vi "Main.vi"(11 "Module Admin":refnum<class "Delacor_lib_QMH_Module Admin.lvclass">) -> ()   [LabVIEW 2019, in "Dashboard.lvlib"]
doc: "This template is based off of the Queued Message Handler design pattern and the Queued Message Handler project template that ships with LabVIEW.\n\nThe main difference is that the queue is private to this module and communication between modules is performed via Broadcast and Request events.\n\nRequest events are wrapped in public API methods and are handled in the Event Handling Loop (EHL) of this VI. Any module can register for Broadcast events sent by this module. The EHL generates messages based on user interface actions.\n\nThe Message Handling Loop (MHL) processes messages generated by the EHL, or by other messages. The messages are string values, so new messages can be added easily to the Message Cases case structure in the MHL. Each message cluster can also provide an optional value for Message Data, which is a variant that can be converted to whatever message-specific data is required.\n_____\nBased on Delacor QMH Project Template 5.0.0.82."
uses:
  Dashboard.lvlib
  <vilib>/Delacor/Delacor QMH/Libraries/Module Admin_class/Delacor_lib_QMH_Module Admin.lvclass
  picam32_LabView_SDK/PICam_lib/types/PicamGatingMode.ctl
  picam32_LabView_SDK/PICam_lib/types/PicamPulse.ctl
  picam32_LabView_SDK/PICam_lib/Ctrls/PicamAdcAnalogGain.ctl
  picam32_LabView_SDK/PICam_lib/Ctrls/PicamAdcQuality.ctl
  picam32_LabView_SDK/PICam_lib/types/PicamSensorTemperatureStatus.ctl
  Module Data--cluster.ctl
  Utility/Types/SetOrGet.ctl
  Update Image Argument--cluster.ctl
  <vilib>/Delacor/Delacor QMH/Libraries/Message Queue_class/Delacor_lib_QMH_Message Queue.lvclass/Delacor_lib_QMH_Message Queue.ctl
  Stop Argument--cluster.ctl
  <vilib>/Utility/miscctls.llb/LVPointTypeDef.ctl
  <vilib>/Delacor/Delacor QMH/Libraries/Module Admin_class/Delacor_lib_QMH_Module Admin.lvclass/Delacor_lib_QMH_Module Admin.ctl
  <vilib>/Delacor/Delacor QMH/Libraries/Message Queue_class/Delacor_lib_QMH_Enqueue Message (Single).vi
  <vilib>/Delacor/Delacor QMH/Libraries/Module Admin_class/Delacor_lib_QMH_Get External Launch.vi
  <vilib>/Utility/error.llb/Error Cluster From Error Code.vi
  <vilib>/ErrorRing/Error Ring.xnode
  <vilib>/Delacor/Delacor QMH/Libraries/Message Queue_class/Delacor_lib_QMH_Message Queue.lvclass
  Spectrometer/Spectrometer.lvlib
  Camera/Camera.lvlib
  FileIO/FileIO.lvlib
  Acquisition Example/Acquisition Example.lvlib
  Notification/Notification.lvlib
  picam32_LabView_SDK/PICam_lib/PICam.lvlib
panel:
  out "Is Running FileIO":bool
  out "Is Running Notification":bool
  in  "Stop Module Notification":bool
  in  "Start Module Notification":bool
  out "Waveform Chart":dbl(graph)
  in  "Acquisition VIs":enum16{"Acquisition Example"}(ring)
  in  "Start Acquisition VI":bool
  in  "Device Tabs":enum32{"Spectrometer", "Camera"}(tab)
  in  "Set Grating":bool
  in  "Set Slit Width":bool
  in  "Grating":i32
  in  "Slit Width":dbl
  in  "Set Wavelength":bool
  in  "Wavelength":dbl
  in  "Tab Control - Camera Parameters":T1(tab)
  in  "IntensifierGain":i32
  in  "EMIccdGain":i32
  in  "CorrectPixelBias":bool
  in  "AdcSpeed":dbl
  in  "AdcBitDepth":i32
  in  "PicamAdcQuality":T2=enum."LowNoise"
  in  "AdcAnalogGain":T3=enum."Medium"
  in  "AdcEMGain":i32
  out "SensorTemperatureStatus":T4
  in  "SensorTemperatureSetPoint":dbl
  out "SensorTemperatureReading":dbl
  out "Temperature Chart":dbl(graph)
  in  "RepetitiveGate":T5
  in  "GatingMode":T6
  in  "V Binning":i32
  in  "V Width":i32
  in  "Vertical":i32
  in  "H Binning":i32
  in  "H Width":i32
  in  "Horizontal":i32
  in  "Acquire Continuously":bool
  in  "Set Accumulations":bool
  in  "Set ROI":bool
  in  "Accumulations":i64 min=0 step=1
  out "Spectrum Graph":u16[][](graph)
  out "CCD Image":u16[][](graph)
  out "Is Running Camera":bool
  in  "Stop Module Camera":bool
  in  "Start Module Camera":bool
  out "Is Running Spectrometer":bool
  in  "Stop Module Spectrometer":bool
  in  "Start Module Spectrometer":bool
  out "Status":string
  # "Module Status"
  # "Spectrometer"
  # "Camera"
  # "Notification"
  # "FileIO"
  # "Data Acquisition"
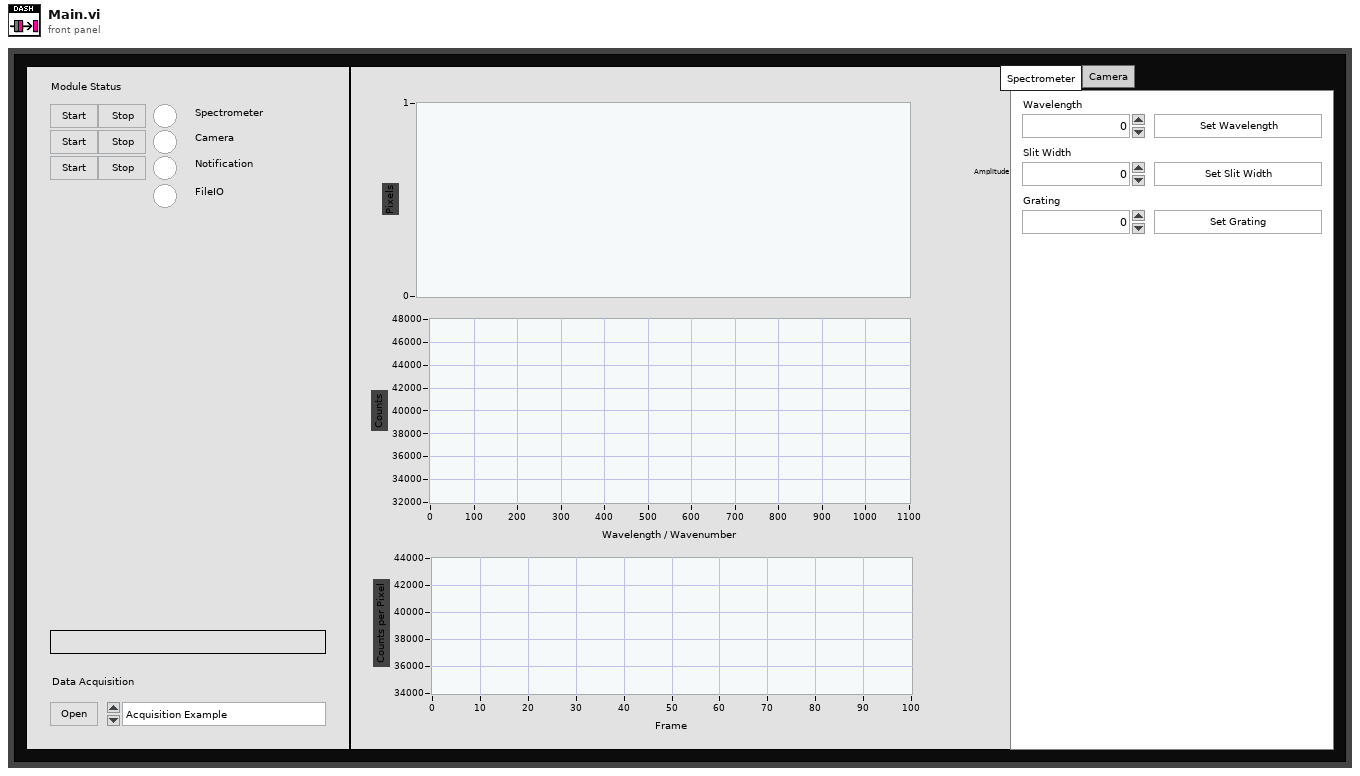
[diagram p1: front panel]
types:
  T1 = enum32{"Intensifier", "ADC", "Gating", "Temperature"}
  T2 = typedef "PICam.lvlib/PicamAdcQuality.ctl" = enum16{"None", "LowNoise", "HighCapacity", "ElectronMultiplied", "HighSpeed"}
  T3 = typedef "PICam.lvlib/PicamAdcAnalogGain.ctl" = enum16{"None", "Low", "Medium", "High"}
  T4 = typedef "PICam.lvlib/PicamSensorTemperatureStatus.ctl" = enum16{"None", "Unlocked", "Locked", "Faulted"}
  T5 = typedef "PICam.lvlib/PicamPulse.ctl" = cluster{"delay":dbl, "width":dbl}
  T6 = typedef "PICam.lvlib/PicamGatingMode.ctl" = enum16{"None", "Repetitive", "Sequential", "Custom", "Disabled"}
  T7 = typedef "Dashboard.lvlib/Request Events--cluster.ctl" = cluster{"Stop Module":refnum<user-event>, "Show Panel":refnum<user-event>, "Hide Panel":refnum<user-event>, "Get Module Execution Status":refnum<user-event>, "Show Diagram":refnum<user-event>}
  T8 = typedef "Notification.lvlib/Broadcast Events--cluster.ctl" = cluster{"Module Did Init":refnum<user-event>, "Status Updated":refnum<user-event>, "Error Reported":refnum<user-event>, "Module Did Stop":refnum<user-event>, "Update Module Execution Status":refnum<user-event>}
  T9 = typedef "Spectrometer.lvlib/Broadcast Events--cluster.ctl" = cluster{"Module Did Init":refnum<user-event>, "Status Updated":refnum<user-event>, "Error Reported":refnum<user-event>, "Module Did Stop":refnum<user-event>, "Update Module Execution Status":refnum<user-event>, "Broadcast Wavelength":refnum<user-event>, "Broadcast Slit Width":refnum<user-event>, "Broadcast Grating":refnum<user-event>}
  T10 = typedef "Camera.lvlib/Broadcast Events--cluster.ctl" = cluster{"Module Did Init":refnum<user-event>, "Status Updated":refnum<user-event>, "Error Reported":refnum<user-event>, "Module Did Stop":refnum<user-event>, "Update Module Execution Status":refnum<user-event>, "Broadcast Image":refnum<user-event>, "Broadcast Exposure Time":refnum<user-event>, "Broadcast Binning":refnum<user-event>, "Broadcast GatingMode":refnum<user-event>, "Broadcast RepetitiveGate":refnum<user-event>, "Broadcast IntensifierStatus":refnum<user-event>, "Broadcast IntensifierGain":refnum<user-event>, "Broadcast EMIccdGainControlMode":refnum<user-event>, "Broadcast EMIccdGain":refnum<user-event>, "Broadcast FloatingPoint Parameter":refnum<user-event>, "Broadcast Integer Parameter":refnum<user-event>, "Broadcast LargeInteger Parameter":refnum<user-event>, "Broadcast Pulse Parameter":refnum<user-event>, "Broadcast SensorTemperatureStatus":refnum<user-event>}
  T11 = typedef "FileIO.lvlib/Broadcast Events--cluster.ctl" = cluster{"Module Did Init":refnum<user-event>, "Status Updated":refnum<user-event>, "Error Reported":refnum<user-event>, "Module Did Stop":refnum<user-event>, "Update Module Execution Status":refnum<user-event>, "File Prepared":refnum<user-event>, "Wrote to File":refnum<user-event>}
  T12 = typedef "Dashboard.lvlib/Module Data--cluster.ctl" = cluster{"Status":string, "Image":u16[][]}
  T13 = enum32{"Invalid", "Standard", "Closed", "Hidden", "Minimized", "Maximized"}
  T14 = typedef "SetOrGet.ctl" = enum16{"Set", "Get"}
  T15 = typedef "Dashboard.lvlib/Update Image Argument--cluster.ctl" = cluster{"Image":u16[][]}
  T16 = enum32{"invalid lock state", "Not Locked", "Locked (No Password)", "Password-protected"}
  T17 = typedef "Dashboard.lvlib/Stop Argument--cluster.ctl" = cluster{"Origin":string, "Exit via Stop Module Req?":bool, "Wait for Module to stop?":bool}
  T18 = typedef "LVPointTypeDef.ctl" = cluster{"Horizontal":i16, "Vertical":i16}
  T19 = typedef "Camera.lvlib/Set GatingMode (Reply Payload)--cluster.ctl" = cluster{"PicamGatingMode":T6, "Set GatingMode_error":errorcluster}
  T20 = typedef "Camera.lvlib/Set RepetitiveGate (Reply Payload)--cluster.ctl" = cluster{"RepetitiveGate":T5, "Set RepetitiveGate_error":errorcluster}
  T21 = typedef "Camera.lvlib/Set Accumulations (Reply Payload)--cluster.ctl" = cluster{"Accumulations":i64, "Set Accumulations_error":errorcluster}
  T22 = cluster{"Horizontal":i32, "H Width":i32, "H Binning":i32, "Vertical":i32, "V Width":i32, "V Binning":i32}
  T23 = typedef "Spectrometer.lvlib/Set Slit Width (Reply Payload)--cluster.ctl" = cluster{"Slit Width (um)":dbl, "Set Slit Width_error":errorcluster}
  T24 = typedef "Spectrometer.lvlib/Set Wavelength (Reply Payload)--cluster.ctl" = cluster{"Wavelength":dbl, "Set Wavelength_error":errorcluster}
  T25 = typedef "Camera.lvlib/SetGet Integer Parameter (Reply Payload)--cluster.ctl" = cluster{"PicamParameter":T26, "Integer Value":i32, "SetGet Integer Parameter_error":errorcluster}
  T26 = typedef "PICam.lvlib/PicamParameter.ctl" = i32
  T27 = typedef "Camera.lvlib/SetGet FloatingPoint Parameter (Reply Payload)--cluster.ctl" = cluster{"FloatingPoint Value":dbl, "PicamParameter":T26, "SetGet FloatingPoint Parameter_error":errorcluster}
  T28 = typedef "Camera.lvlib/ROI--cluster.ctl" = cluster{"_Horizontal":i32, "_Horizontal Width":i32, "_Horizontal Binning":i32, "_Vertical":i32, "_Vertical Width":i32, "_Vertical Binning":i32}
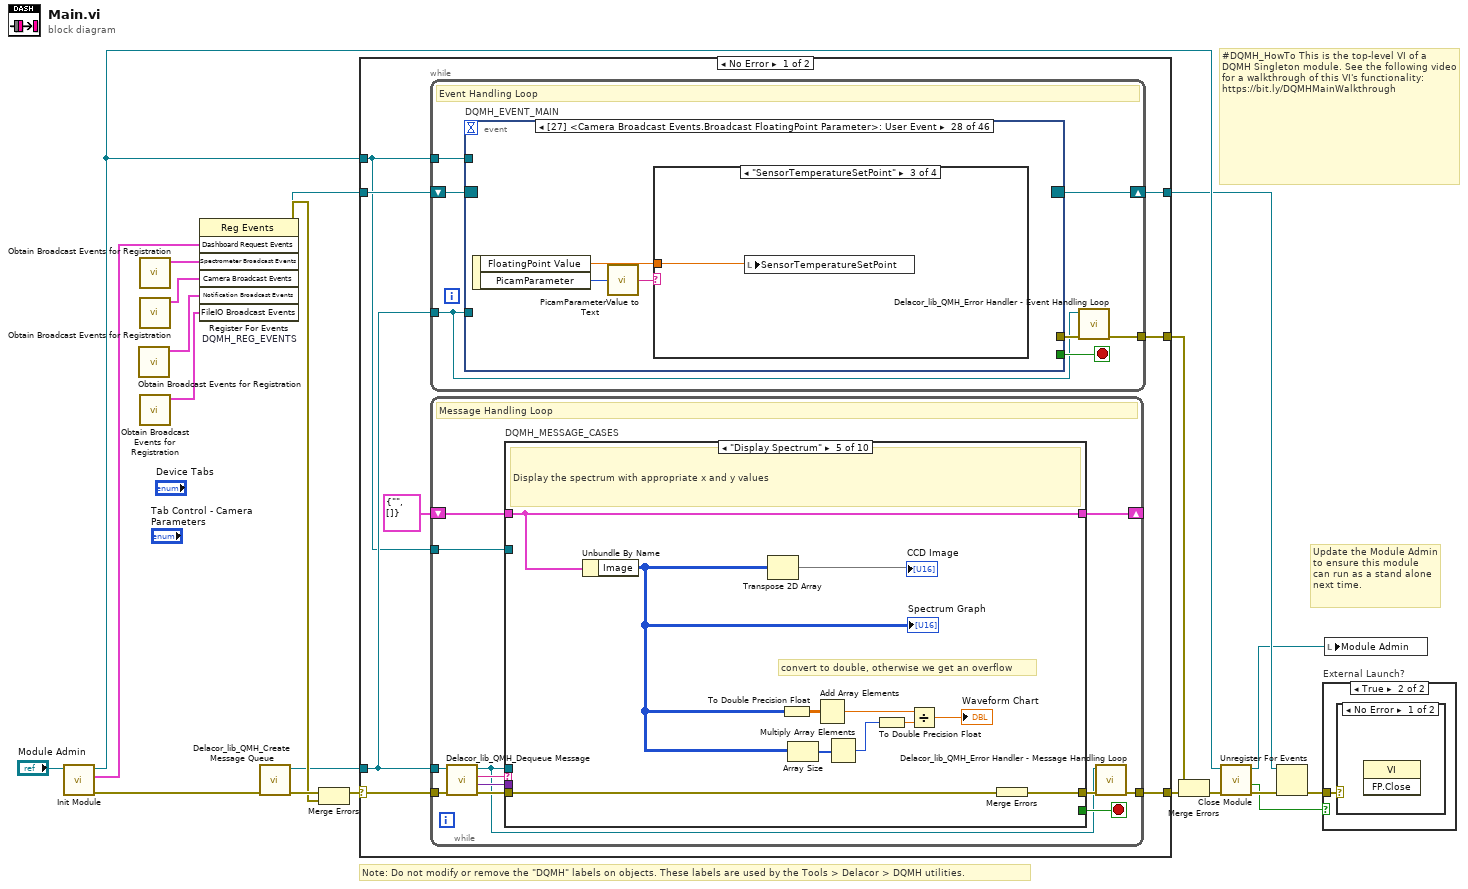
[diagram p0: block diagram]
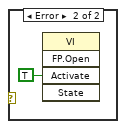
[diagram p3: hidden frame]
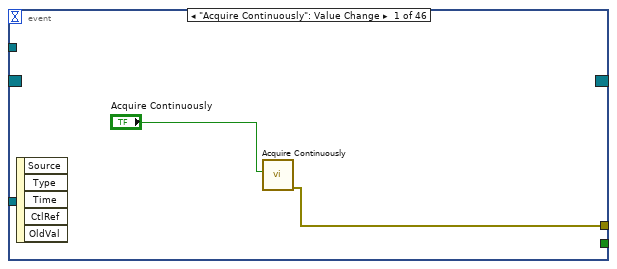
[diagram p4: hidden frame]
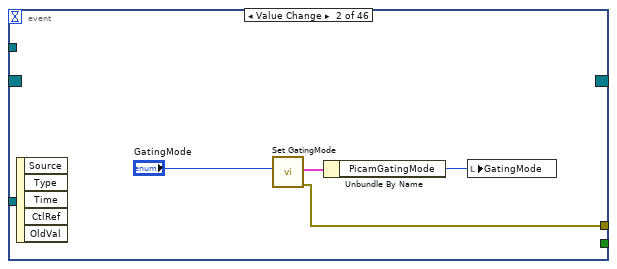
[diagram p5: hidden frame]
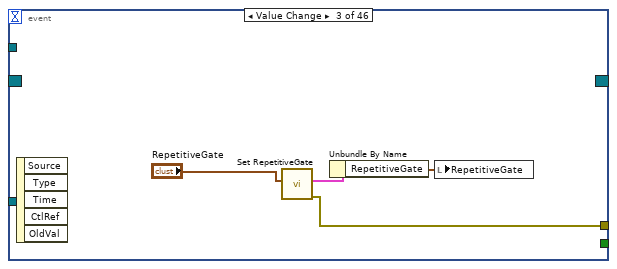
[diagram p6: hidden frame]
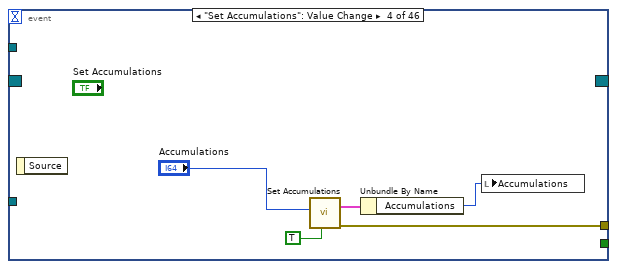
[diagram p7: hidden frame]
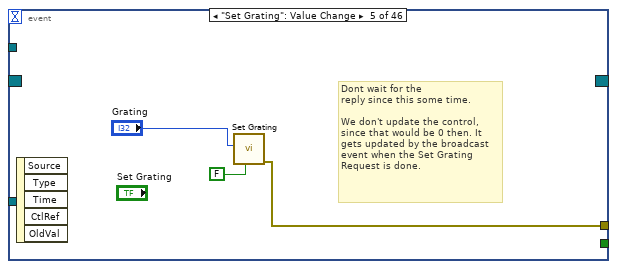
[diagram p8: hidden frame]
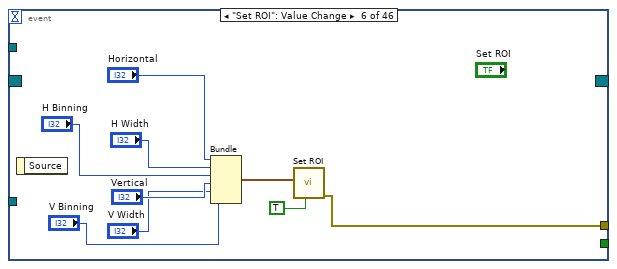
[diagram p9: hidden frame]
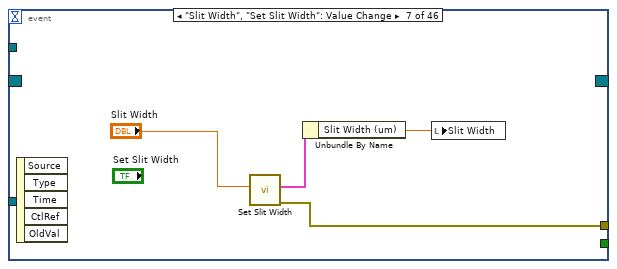
[diagram p10: hidden frame]
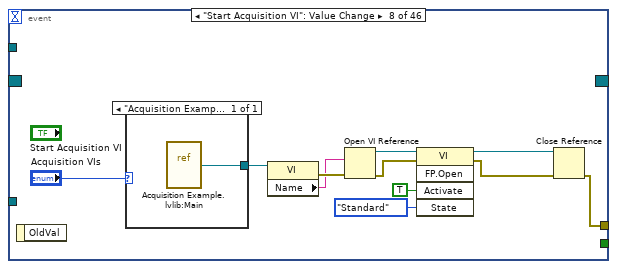
[diagram p11: hidden frame]
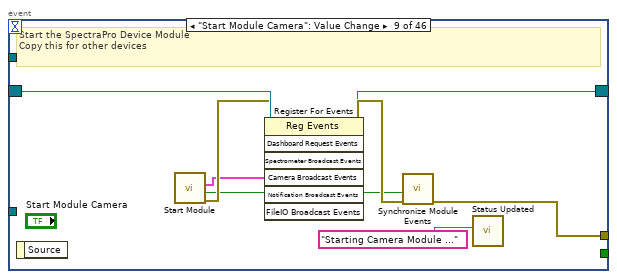
[diagram p12: hidden frame]
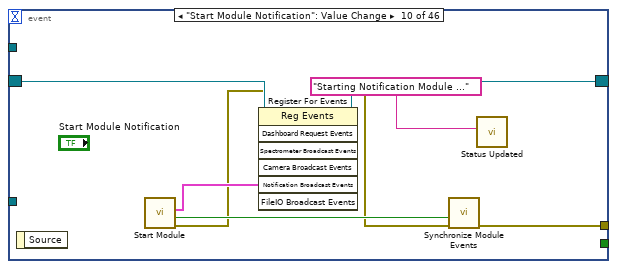
[diagram p13: hidden frame]
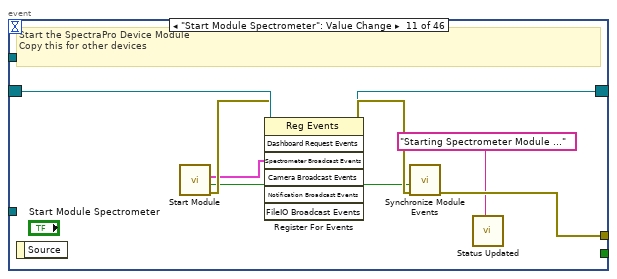
[diagram p14: hidden frame]
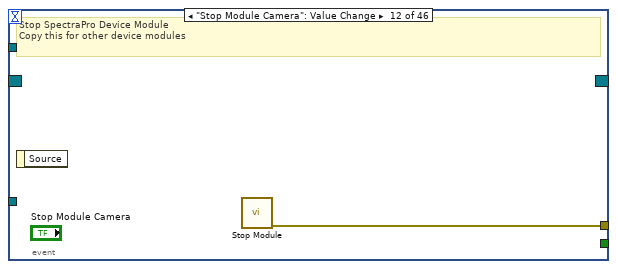
[diagram p15: hidden frame]
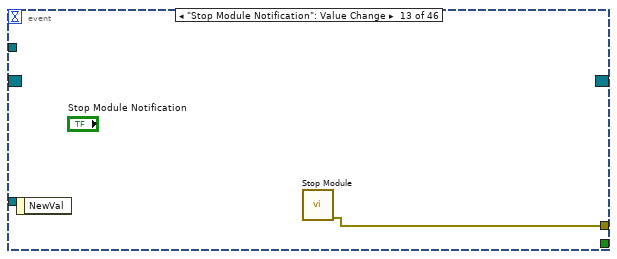
[diagram p16: hidden frame]
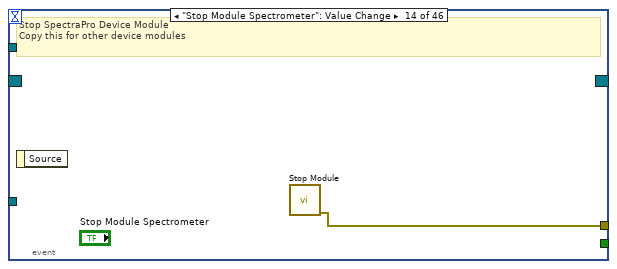
[diagram p17: hidden frame]
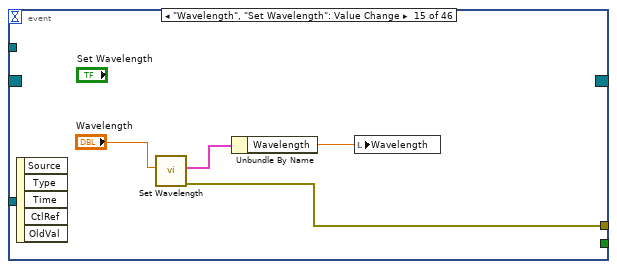
[diagram p18: hidden frame]
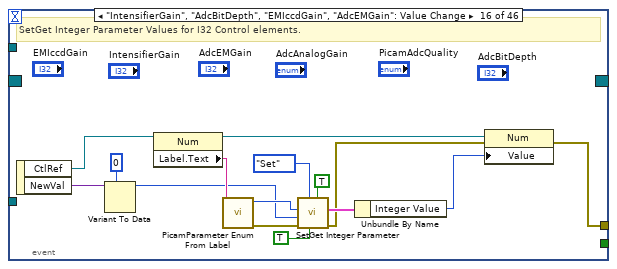
[diagram p19: hidden frame]
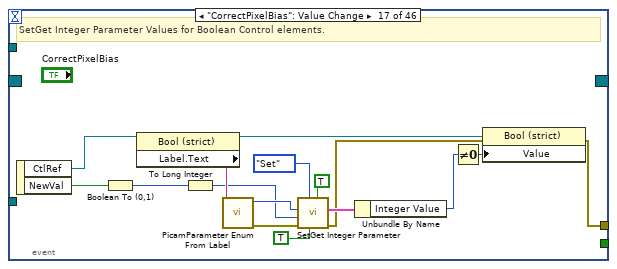
[diagram p20: hidden frame]
diagram:
  # "#DQMH_HowTo This is the top-level VI of a DQMH Singleton module. See the following video for a walkthrough of this VI's functionality: https://bit.ly/DQMHMainWalkthrough"
  # "Note: Do not modify or remove the \"DQMH\" labels on objects. These labels are used by the Tools > Delacor > DQMH utilities."
  # "Update the Module Admin to ensure this module can run as a stand alone next time."
  n1 = call "Init Module.vi"("Singleton Module Admin in"="Module Admin") -> ("error out"=w20:errorcluster, "Dashboard Request Events"=w9:T7, "Singleton Module Admin out"=w12:refnum<class "Delacor_lib_QMH_Module Admin.lvclass">)  [unwired: 8 in]
  n2 = call "Obtain Broadcast Events for Registration.vi"() -> ("Notification Broadcast Events"=w1:T8)  [unwired: 9 in, 2 out]
  n3 = call "Obtain Broadcast Events for Registration.vi"() -> ("Spectrometer Broadcast Events"=w4:T9)  [unwired: 9 in, 2 out]
  n4 = call "Obtain Broadcast Events for Registration.vi"() -> ("Camera Broadcast Events"=w3:T10)  [unwired: 9 in, 2 out]
  n5 = call "Obtain Broadcast Events for Registration.vi"() -> ("FileIO Broadcast Events"=w2:T11)  [unwired: 9 in, 2 out]
  n6 = register-events "DQMH_REG_EVENTS"(w9, w4, w3, w1, w2) -> (reference out=w10:refnum<event-registration>, error out=w13:errorcluster)  [unwired: 2 in]
  n7 = call <vilib>:"Delacor_lib_QMH_Create Message Queue.vi"("error in (no error)"=w20) -> ("error out"=w15:errorcluster, "Message Queue"=w8:refnum<class "Delacor_lib_QMH_Message Queue.lvclass">)  [unwired: 9 in]
  n8 = Merge Errors(w15, w13) -> (w14:errorcluster)
  n9 = case shown="No Error" w14 {
    selector: w14 -> [w27 w357]
    tunnel: [w29 w356] -> w21
    tunnel: [w26 w362] -> w11
    tunnel: w10 -> [w24 w362]
    tunnel: w8 -> [w23 w355]
    tunnel: [w28 _] -> w18
    tunnel: w12 -> [w22 w358]
    frame No Error {
      n10 = while {
        tunnel: w23 -> [w30]
        shift-right: [w33] -> w26
        shift-left: w24 -> [w34]
        tunnel: [w35] -> w28
        tunnel: w22 -> [w31]
        stop <- w32 stop-if-true
        # "Event Handling Loop"
        n11 = event "DQMH_EVENT_MAIN" shown="[27] <Camera Broadcast Events.Broadcast FloatingPoint Parameter>: User Event" {
          selector: w34 -> [_ _ _ _ _ _ _ _ w87 w93 w103 _ _ _ _ _ _ _ _ _ _ _ _ _ _ _ _ _ _ _ _ _ _ _ _ _ _ _ _ _ _ _ _ _ _ _]
          dyn-events: [_ _ _ _ _ _ _ _ w84 w92 w97 _ _ _ _ _ _ _ _ _ _ _ _ _ _ _ _ _ _ _ _ _ _ _ _ _ _ _ _ _ _ _ _ _ _ _] -> w33
          timeout: _ -> [_ _ _ _ _ _ _ _ _ _ _ _ _ _ _ _ _ _ _ _ _ _ _ _ _ _ _ _ _ _ _ _ _ _ _ _ _ _ _ _ _ _ _ _ _ _]
          tunnel: [_ _ _ _ _ _ _ _ _ _ _ _ _ _ _ _ _ _ _ _ _ _ _ _ _ _ _ _ _ _ _ _ TRUE ("Discard?") _ _ _ _ _ _ _ _ _ _ _ _ _] -> w32
          tunnel: w30 -> [_ _ _ _ _ _ _ _ _ _ _ _ _ _ _ _ _ _ _ _ _ w173 _ _ _ _ _ _ _ _ _ _ w215 _ _ _ _ _ _ _ _ _ _ _ _ w234]
          tunnel: [w37 w41 w45 w50 w53 w63 w66 w74 w82 w94 w101 w104 w105 w106 w109 w113 w129 w144 _ _ _ w174 _ _ _ _ _ _ w194 _ _ _ w218 _ _ _ _ _ _ _ _ _ _ _ _ w236] -> w36
          tunnel: w31 -> [_ _ _ _ _ _ _ _ _ _ _ _ _ _ _ _ _ _ _ _ _ _ _ _ _ _ _ _ _ _ _ _ _ _ _ _ _ _ _ _ _ _ _ _ _ _]
          event "Acquire Continuously": Value Change {
            n12 = event-data() -> ()  [unwired: 1 in, 5 out]
            n13 = call "Acquire Continuously.vi"("Acquire Continuously"="Acquire Continuously") -> ("error out"=w37:errorcluster)  [unwired: 10 in]
          }
          event Value Change {
            n14 = event-data() -> ()  [unwired: 1 in, 5 out]
            n15 = call "Set GatingMode.vi"("PicamGatingMode"="GatingMode") -> ("error out"=w41:errorcluster, "Reply Payload"=w40:T19)  [unwired: 8 in, 1 out]
            n16 = Unbundle By Name(w40) -> ("PicamGatingMode"=w39:T6)
            n17 = local write "GatingMode"(w39) -> ()
          }
          event Value Change {
            n18 = event-data() -> ()  [unwired: 1 in, 5 out]
            n19 = call "Set RepetitiveGate.vi"("RepetitiveGate"="RepetitiveGate") -> ("error out"=w45:errorcluster, "Reply Payload"=w44:T20)  [unwired: 8 in, 1 out]
            n20 = Unbundle By Name(w44) -> ("RepetitiveGate"=w43:T5)
            n21 = local write "RepetitiveGate"(w43) -> ()
          }
          event "Set Accumulations": Value Change {
            n22 = event-data() -> ()  [unwired: 1 in, 1 out]
            n23 = call "Set Accumulations.vi"("wait for reply (T)"=TRUE, "Accumulations"="Accumulations") -> ("error out"=w50:errorcluster, "Reply Payload"=w48:T21)  [unwired: 7 in, 1 out]
            n24 = Unbundle By Name(w48) -> ("Accumulations"=w47:i64)
            n25 = local write "Accumulations"(w47) -> ()
          }
          event "Set Grating": Value Change {
            # "Dont wait for the\nreply since this some time.\n\nWe don't update the control,\nsince that would be 0 then. It\ngets updated by the broadcast\nevent when the Set Grating\nRequest is done."
            n26 = event-data() -> ()  [unwired: 1 in, 5 out]
            n27 = call "Set Grating.vi"("wait for reply (T)"=FALSE, "Grating ID"="Grating") -> ("error out"=w53:errorcluster)  [unwired: 7 in, 2 out]
          }
          event "Set ROI": Value Change {
            n28 = event-data() -> ()  [unwired: 1 in, 1 out]
            n29 = Bundle("Horizontal"="Horizontal", "H Width"="H Width", "H Binning"="H Binning", "Vertical"="Vertical", "V Width"="V Width", "V Binning"="V Binning") -> (w55:T22)  [unwired: 1 in]
            n30 = call "Set ROI.vi"("wait for reply (T)"=TRUE, "ROI"=w55) -> ("error out"=w63:errorcluster)  [unwired: 7 in, 2 out]
          }
          event "Slit Width", "Set Slit Width": Value Change {
            n31 = event-data() -> ()  [unwired: 1 in, 5 out]
            n32 = call "Set Slit Width.vi"("Slit Width (um)"="Slit Width") -> ("error out"=w66:errorcluster, "Reply Payload"=w65:T23)  [unwired: 8 in, 1 out]
            n33 = Unbundle By Name(w65) -> ("Slit Width (um)"=w64:dbl)
            n34 = local write "Slit Width"(w64) -> ()
          }
          event "Start Acquisition VI": Value Change {
            n35 = event-data() -> ()  [unwired: 1 in, 1 out]
            n36 = case shown="\"Acquisition Example\", Default" "Acquisition VIs" {
              tunnel: [w79] -> w77
              frame "Acquisition Example", Default {
                n37 = vi-ref "Acquisition Example.lvlib:Main.vi"() -> (w79:refnum<vi>)
              }
            }
            n38 = property class="VI"(reference=w77) -> (error out=w76:errorcluster, "Name"=w75:string)  [unwired: 1 in, 1 out]
            n39 = Open VI Reference(vi path=w75, error in (no error)=w76) -> (vi reference=w73:refnum<vi>, error out=w70:errorcluster)  [unwired: 4 in]
            n40 = invoke class="VI" method="FP.Open"(reference=w73, error in=w70, "Activate"=TRUE ("Activate?"), "State"=T13."Standard") -> (reference out=w71:refnum<vi>, error out=w69:errorcluster)  [unwired: 1 in, 3 out]
            n41 = Close Reference(reference=w71, error in (no error)=w69) -> (error out=w74:errorcluster)
          }
          event "Start Module Camera": Value Change {
            # "Start the SpectraPro Device Module\nCopy this for other devices"
            n42 = event-data() -> ()  [unwired: 1 in, 1 out]
            n43 = call "Start Module.vi"() -> ("error out"=w83:errorcluster, "Wait for Event Sync?"=w80:bool, "Camera Broadcast Events"=w81:T10)  [unwired: 8 in, 1 out]
            n44 = register-events(reference=w87, error in=w83, w81) -> (reference out=w84:refnum<event-registration>, error out=w86:errorcluster)  [unwired: 4 in]
            n45 = call "Synchronize Module Events.vi"("error in (no error)"=w86, "Wait for Event Sync?"=w80) -> ("error out"=w82:errorcluster)  [unwired: 9 in]
            n46 = call "Status Updated.vi"("Status"="Starting Camera Module ...") -> ()  [unwired: 10 in, 1 out]
          }
          event "Start Module Notification": Value Change {
            n47 = event-data() -> ()  [unwired: 1 in, 1 out]
            n48 = call "Start Module.vi"() -> ("error out"=w90:errorcluster, "Wait for Event Sync?"=w95:bool, "Notification Broadcast Events"=w91:T8)  [unwired: 8 in, 1 out]
            n49 = register-events(reference=w93, error in=w90, w91) -> (reference out=w92:refnum<event-registration>, error out=w89:errorcluster)  [unwired: 4 in]
            n50 = call "Synchronize Module Events.vi"("error in (no error)"=w89, "Wait for Event Sync?"=w95) -> ("error out"=w94:errorcluster)  [unwired: 9 in]
            n51 = call "Status Updated.vi"("Status"="Starting Notification Module ...") -> ()  [unwired: 10 in, 1 out]
          }
          event "Start Module Spectrometer": Value Change {
            # "Start the SpectraPro Device Module\nCopy this for other devices"
            n52 = event-data() -> ()  [unwired: 1 in, 1 out]
            n53 = call "Start Module.vi"() -> ("error out"=w102:errorcluster, "Wait for Event Sync?"=w99:bool, "Spectrometer Broadcast Events"=w96:T9)  [unwired: 8 in, 1 out]
            n54 = register-events(reference=w103, error in=w102, w96) -> (reference out=w97:refnum<event-registration>, error out=w100:errorcluster)  [unwired: 4 in]
            n55 = call "Synchronize Module Events.vi"("error in (no error)"=w100, "Wait for Event Sync?"=w99) -> ("error out"=w101:errorcluster)  [unwired: 9 in]
            n56 = call "Status Updated.vi"("Status"="Starting Spectrometer Module ...") -> ()  [unwired: 10 in, 1 out]
          }
          event "Stop Module Camera": Value Change {
            # "Stop SpectraPro Device Module\nCopy this for other device modules"
            n57 = event-data() -> ()  [unwired: 1 in, 1 out]
            n58 = call "Stop Module.vi"() -> ("error out"=w104:errorcluster)  [unwired: 11 in]
          }
          event "Stop Module Notification": Value Change {
            n59 = event-data() -> ()  [unwired: 1 in, 1 out]
            n60 = call "Stop Module.vi"() -> ("error out"=w105:errorcluster)  [unwired: 11 in]
          }
          event "Stop Module Spectrometer": Value Change {
            # "Stop SpectraPro Device Module\nCopy this for other device modules"
            n61 = event-data() -> ()  [unwired: 1 in, 1 out]
            n62 = call "Stop Module.vi"() -> ("error out"=w106:errorcluster)  [unwired: 11 in]
          }
          event "Wavelength", "Set Wavelength": Value Change {
            n63 = event-data() -> ()  [unwired: 1 in, 5 out]
            n64 = call "Set Wavelength.vi"("Wavelength"="Wavelength") -> ("error out"=w109:errorcluster, "Reply Payload"=w108:T24)  [unwired: 8 in, 1 out]
            n65 = Unbundle By Name(w108) -> ("Wavelength"=w107:dbl)
            n66 = local write "Wavelength"(w107) -> ()
          }
          event "IntensifierGain", "AdcBitDepth", "EMIccdGain", "AdcEMGain": Value Change {
            # "SetGet Integer Parameter Values for I32 Control elements."
            n67 = event-data() -> ("CtlRef"=w122:refnum<vi>, "NewVal"=w125:variant)  [unwired: 1 in]
            n68 = Variant To Data(type=0, Variant=w125) -> (data=w111:i32)  [unwired: 1 in, 1 out]
            n69 = property class="Num"(reference=w122) -> (reference out=w117:refnum<vi>, "Label.Text"=w121:string)  [unwired: 1 in, 1 out]
            n70 = call "PicamParameter Enum From Label.vi"("String"=w121) -> ("error out"=w123:errorcluster, "Numeric"=w124:i32)  [unwired: 9 in]
            n71 = call "SetGet Integer Parameter.vi"("Broadcast"=TRUE, "wait for reply (T)"=TRUE, "SetOrGet"=SetOrGet."Set", "error in (no error)"=w123, "Integer Value"=w111, "PicamParameter"=w124) -> ("error out"=w114:errorcluster, "Reply Payload"=w116:T25)  [unwired: 3 in, 1 out]
            n72 = Unbundle By Name(w116) -> ("Integer Value"=w115:i32)
            n73 = property class="Num"(reference=w117, error in=w114, "Value"=w115) -> (error out=w113:errorcluster)  [unwired: 1 out]
          }
          event "CorrectPixelBias": Value Change {
            # "SetGet Integer Parameter Values for Boolean Control elements."
            n74 = event-data() -> ("CtlRef"=w138:refnum<vi>, "NewVal"=w141:bool)  [unwired: 1 in]
            n75 = Boolean To (0,1)(Boolean=w141) -> (0, 1=w128:i16)
            n76 = property class="Bool (strict)"(reference=w138) -> (reference out=w133:refnum<vi>, "Label.Text"=w137:string)  [unwired: 1 in, 1 out]
            n77 = To Long Integer(number=w128) -> (32bit integer=w127:i32)
            n78 = call "PicamParameter Enum From Label.vi"("String"=w137) -> ("error out"=w139:errorcluster, "Numeric"=w140:i32)  [unwired: 9 in]
            n79 = call "SetGet Integer Parameter.vi"("Broadcast"=TRUE, "wait for reply (T)"=TRUE, "SetOrGet"=SetOrGet."Set", "error in (no error)"=w139, "Integer Value"=w127, "PicamParameter"=w140) -> ("error out"=w130:errorcluster, "Reply Payload"=w132:T25)  [unwired: 3 in, 1 out]
            n80 = Unbundle By Name(w132) -> ("Integer Value"=w131:i32)
            n81 = Not Equal To 0?(x=w131) -> (x != 0?=w126:bool)
            n82 = property class="Bool (strict)"(reference=w133, error in=w130, "Value"=w126) -> (error out=w129:errorcluster)  [unwired: 1 out]
          }
          event "AdcSpeed", "SensorTemperatureSetPoint": Value Change {
            # "SetGet FloatingPoint Parameter Values"
            n83 = event-data() -> ("CtlRef"=w153:refnum<vi>, "NewVal"=w156:dbl)  [unwired: 1 in]
            n84 = Variant To Data(type=0.0, Variant=w156) -> (data=w142:dbl)  [unwired: 1 in, 1 out]
            n85 = property class="DigNum (strict)"(reference=w153) -> (reference out=w148:refnum<vi>, "Label.Text"=w152:string)  [unwired: 1 in, 1 out]
            n86 = call "PicamParameter Enum From Label.vi"("String"=w152) -> ("error out"=w154:errorcluster, "Numeric"=w155:i32)  [unwired: 9 in]
            n87 = call "SetGet FloatingPoint Parameter.vi"("Broadcast"=TRUE, "wait for reply (T)"=TRUE, "SetOrGet"=SetOrGet."Set", "error in (no error)"=w154, "FloatingPoint Value"=w142, "PicamParameter"=w155) -> ("error out"=w145:errorcluster, "Reply Payload"=w147:T27)  [unwired: 3 in, 1 out]
            n88 = Unbundle By Name(w147) -> ("FloatingPoint Value"=w146:dbl)
            n89 = property class="DigNum (strict)"(reference=w148, error in=w145, "Value"=w146) -> (error out=w144:errorcluster)  [unwired: 1 out]
          }
          event User Event {
            # "#TODO: The broadcast event is named incorrectly"
            n90 = event-data() -> ("ROI"=w163:T28)  [unwired: 1 in]
            n91 = Unbundle By Name(w163) -> ("_Horizontal"=w162:i32, "_Horizontal Width"=w161:i32, "_Horizontal Binning"=w160:i32, "_Vertical"=w159:i32, "_Vertical Width"=w158:i32, "_Vertical Binning"=w157:i32)
            n92 = local write "Horizontal"(w162) -> ()
            n93 = local write "H Binning"(w160) -> ()
            n94 = local write "V Binning"(w157) -> ()
            n95 = local write "H Width"(w161) -> ()
            n96 = local write "V Width"(w158) -> ()
            n97 = local write "Vertical"(w159) -> ()
          }
          event User Event {
            # "#TODO The broadcast event is named incorrectly"
            n98 = event-data() -> ("Accumulations"=w164:i64)  [unwired: 1 in]
            n99 = local write "Accumulations"(w164) -> ()
          }
          event User Event {
            n100 = event-data() -> ("PicamGatingMode"=w165:T6)  [unwired: 1 in]
            n101 = local write "GatingMode"(w165) -> ()
          }
          event User Event {
            n102 = event-data() -> ("Image"=w168:u16[][])  [unwired: 1 in]
            n103 = Bundle(cluster=T15 {"Image"=[]} ("Update Image Argument"), "Image"=w168) -> (w166:T15)
            n104 = call-poly <vilib>:"Delacor_lib_QMH_Enqueue Message (poly).vi"("Message Data"=w166, "Message"="Update Spectrum", "Message Queue in"=w173) -> ("error out"=w170:errorcluster, "Message Queue out"=w171:refnum<class "Delacor_lib_QMH_Message Queue.lvclass">)  [unwired: 7 in]
            n105 = call-poly <vilib>:"Delacor_lib_QMH_Enqueue Message (poly).vi"("error in (no error)"=w170, "Message"="Display Spectrum", "Message Queue in"=w171) -> ("error out"=w174:errorcluster)  [unwired: 7 in, 1 out]
          }
          event User Event {
            n106 = event-data() -> ("RepetitiveGate"=w175:T5)  [unwired: 1 in]
            n107 = local write "RepetitiveGate"(w175) -> ()
          }
          event User Event {
            n108 = event-data() -> ("Init?"=→"Is Running Camera":bool)  [unwired: 1 in, 1 out]
          }
          event User Event {
            n109 = event-data() -> ()  [unwired: 1 in, 5 out]
            n110 = local write "Is Running Camera"(FALSE ("Is Running SpectraPro")) -> ()
          }
          event User Event {
            n111 = event-data() -> ("Running?"=w178:bool)  [unwired: 1 in]
            n112 = local write "Is Running Camera"(w178) -> ()
          }
          event User Event {
            n113 = event-data() -> ("Integer Value"=w181:i32, "PicamParameter"=w180:T26)  [unwired: 1 in]
            n114 = call "PicamParameterValue to Text.vi"("ParameterValue"=w180) -> ("Parameter Text"=w179:string)
            n115 = case shown="\"SensorTemperatureStatus\"" w179 {
              tunnel: w181 -> [_ w182 w183 w184 w185 w186]
              frame "0", Default {
              }
              frame "AdcAnalogGain" {
                n116 = local write "AdcAnalogGain"(w182) -> ()
              }
              frame "AdcEMGain" {
                n117 = local write "AdcEMGain"(w183) -> ()
              }
              frame "IntensifierGain" {
                n118 = local write "IntensifierGain"(w184) -> ()
              }
              frame "EMIccdGain" {
                n119 = local write "EMIccdGain"(w185) -> ()
              }
              frame "SensorTemperatureStatus" {
                "SensorTemperatureStatus" <- w186
              }
            }
          }
          event User Event {
            n120 = event-data() -> ("FloatingPoint Value"=w189:dbl, "PicamParameter"=w188:T26)  [unwired: 1 in]
            n121 = call "PicamParameterValue to Text.vi"("ParameterValue"=w188) -> ("Parameter Text"=w187:string)
            n122 = case shown="\"SensorTemperatureSetPoint\"" w187 {
              tunnel: w189 -> [_ w190 w191 w192]
              frame "0", Default {
              }
              frame "SensorTemperatureReading" {
                "SensorTemperatureReading" <- w190
                "Temperature Chart" <- w190
              }
              frame "SensorTemperatureSetPoint" {
                n123 = local write "SensorTemperatureSetPoint"(w191) -> ()
              }
              frame "AdcSpeed" {
                n124 = local write "AdcSpeed"(w192) -> ()
              }
            }
          }
          event User Event {
            # "Another Module called the \"Get Module Execution Status\" API Method."
            n125 = event-data() -> ()  [unwired: 1 in, 1 out]
            n126 = call "Update Module Execution Status.vi"("Running?"=TRUE) -> ("error out"=w194:errorcluster)  [unwired: 10 in]
          }
          event User Event {
            # "Hide the panel of this VI, and send a status updated message to let listeners know."
            # "Another Module called the \"Hide Panel\" API Method."
            n127 = event-data() -> ()  [unwired: 1 in, 1 out]
            n128 = control-ref of="This VI"() -> (w196:refnum<vi>)
            n129 = call "Hide VI Panel.vi"("VI"=w196) -> ()  [unwired: 10 in, 1 out]
            n130 = call "Status Updated.vi"("Status"="Panel hidden." ("format string")) -> ()  [unwired: 10 in, 1 out]
          }
          event User Event {
            # "Another Module called the \"Show Diagram\" API Method. This event is used for debugging."
            n131 = event-data() -> ()  [unwired: 1 in, 1 out]
            n132 = disable-structure shown="RUN_TIME_ENGINE==False" {
              frame condition #0 (active) {
                # "functionality not available in exe"
                n133 = invoke class="VI" method="Lock State.Get"() -> (error out=w202:errorcluster, "Get Lock State"=w201:T16, "pwd in cache"=w198:bool)  [unwired: 4 in, 1 out]
                n134 = Equal?(x=T16."Password-protected", y=w201) -> (x = y?=w199:bool)
                n135 = Compound Arithmetic op=AND(w199, invert w198) -> (w197:bool)
                n136 = case shown="False" w197 {
                  tunnel: w202 -> [w205 _]
                  frame False {
                    n137 = property class="VI"(error in=w205, "BDWin.Open"=TRUE ("Block Diagram Window:Open")) -> ()  [unwired: 1 in, 2 out]
                    n138 = call "Status Updated.vi"("Status"="Block Diagram shown." ("format string")) -> ()  [unwired: 10 in, 1 out]
                  }
                  frame True {
                    # "Password-protected VI, and the password is not in the cache. Do not show the diagram."
                  }
                }
              }
              frame condition #1 {
              }
            }
          }
          event User Event {
            # "Show the panel of this VI, and send a status updated message to let listeners know."
            # "Another Module called the \"Show Panel\" API Method."
            n139 = event-data() -> ()  [unwired: 1 in, 1 out]
            n140 = control-ref of="This VI"() -> (w207:refnum<vi>)
            n141 = call "Open VI Panel.vi"("VI"=w207) -> ()  [unwired: 10 in, 1 out]
            n142 = call "Status Updated.vi"("Status"="Panel shown." ("format string")) -> ()  [unwired: 10 in, 1 out]
          }
          event User Event {
            # "The Stop Module Event can get fired from the Exit message in the MHL. The queue gets destroyed in that case. If the queue no longer exists, the Enqueue Exit as a priority message will return error 1. It is safe to ignore, because the module is already exiting."
            # "Another Module called the \"Stop Module\" API Method  or the Message Handling Loop below."
            n143 = event-data() -> ("Origin"=w214:string, "Exit via Stop Module Req?"=w210:bool, "Wait for Module to stop?"=w209:bool)  [unwired: 1 in]
            n144 = local write "Status"(w214) -> ()
            n145 = Bundle By Name(cluster=T17 {"Origin"="", "Exit via Stop Module Req?"=FALSE, "Wait for Module to stop?"=FALSE} ("Stop Argument"), "Exit via Stop Module Req?"=w210, "Wait for Module to stop?"=w209) -> (w208:T17)
            n146 = call-poly <vilib>:"Delacor_lib_QMH_Enqueue Message (poly).vi"("Priority Message? (F)"=TRUE, "Message Data"=w208, "Message"="Exit", "Message Queue in"=w215) -> ("error out"=w219:errorcluster)  [unwired: 6 in, 1 out]
            n147 = call <vilib>:"Clear Errors.vi"("error in (no error)"=w219, "specific error code to clear (0: all)"=1) -> ("error out"=w218:errorcluster)  [unwired: 4 in, 1 out]
          }
          event User Event {
            n148 = event-data() -> ("Init?"=→"Is Running Notification":bool)  [unwired: 1 in, 4 out]
          }
          event User Event {
            n149 = event-data() -> ()  [unwired: 1 in, 5 out]
            n150 = local write "Is Running Notification"(FALSE ("Is Running Notification")) -> ()
          }
          event User Event {
            # "The FileIO Module should always be running.  Let the LED blink when it stops."
            n151 = event-data() -> ()  [unwired: 1 in, 5 out]
            "Is Running FileIO" <- FALSE ("Is Running FileIO")
          }
          event User Event {
            n152 = event-data() -> ("Running?"=w223:bool)  [unwired: 1 in]
            n153 = local write "Is Running Spectrometer"(w223) -> ()
          }
          event User Event {
            n154 = event-data() -> ("Running?"=w224:bool)  [unwired: 1 in]
            n155 = local write "Is Running FileIO"(w224) -> ()
          }
          event User Event {
            n156 = event-data() -> ("Grating ID"=w225:u32)  [unwired: 1 in, 4 out]
            n157 = local write "Grating"(w225) -> ()
          }
          event User Event {
            n158 = event-data() -> ("Slit Width (um)"=w226:dbl)  [unwired: 1 in, 4 out]
            n159 = local write "Slit Width"(w226) -> ()
          }
          event User Event {
            n160 = event-data() -> ("Wavelength"=w227:dbl)  [unwired: 1 in]
            n161 = local write "Wavelength"(w227) -> ()
          }
          event User Event {
            n162 = event-data() -> ("Init?"=→"Is Running Spectrometer":bool)  [unwired: 1 in, 1 out]
          }
          event User Event {
            n163 = event-data() -> ()  [unwired: 1 in, 5 out]
            n164 = local write "Is Running Spectrometer"(FALSE ("Is Running SpectraPro")) -> ()
          }
          event User Event {
            # "A sub-module updated it's status"
            n165 = event-data() -> ("Status"=w230:string)  [unwired: 1 in]
            n166 = local write "Status"(w230) -> ()
          }
          event User Event {
            n167 = event-data() -> ("Running?"=w231:bool)  [unwired: 1 in]
            n168 = local write "Is Running Spectrometer"(w231) -> ()
          }
          event Panel Close? {
            w235 = TRUE  # Discard the event, the MHL is responsible for closing and stopping this VI.
            # "Stop this module regardless if it was launched externally or not.\nIt should be started by the Launcher.vi anyhow."
            # "Hide the panel or send the 'Exit' message if the user clicks the 'X' on the module main VI panel."
            n169 = event-data() -> ()  [unwired: 1 in, 1 out]
            n170 = call-poly <vilib>:"Delacor_lib_QMH_Enqueue Message (poly).vi"("Priority Message? (F)"=TRUE, "Message"="Exit", "Message Queue in"=w234) -> ("error out"=w236:errorcluster)  [unwired: 7 in, 1 out]
            n171 = event-data("Discard?"=w235) -> ()  [unwired: 1 in, 1 out]
          }
        }
        n172 = call-dynamic "Delacor_lib_QMH_Error Handler - Event Handling Loop.vi"("error in (no error)"=w36, "Message Queue in"=w30) -> ("dup error in"=w35:errorcluster)  [unwired: 8 in, 1 out]
      }
      n173 = while {
        tunnel: w23 -> [w239]
        shift-right: [w243] -> _
        shift-left: T12 {"Status"="", "Image"=[]} ("Data Cluster") -> [w244]
        tunnel: w27 -> [w247]
        tunnel: [w245] -> w29
        tunnel: w22 -> [w237]
        stop <- w242 stop-if-true
        # "Message Handling Loop"
        n174 = call-dynamic "Delacor_lib_QMH_Dequeue Message.vi"("error in (no error)"=w247, "Message Queue in"=w239) -> ("error out"=w246:errorcluster, "Message Data"=w240:variant, "Message"=w241:string, "Message Queue out"=w238:refnum<class "Delacor_lib_QMH_Message Queue.lvclass">)  [unwired: 6 in]
        n175 = case "DQMH_MESSAGE_CASES" shown="\"Display Spectrum\"" w241 {
          selector: w241 -> [_ _ _ _ _ _ _ _ _ w342]
          tunnel: w238 -> [_ _ _ _ _ _ _ w313 w334 _]
          tunnel: w246 -> [w267 w271 w274 w283 w294 w296 w301 w319 w340 w344]
          tunnel: [w249 w271 w273 w282 w293 w296 w300 w309 w337 w345] -> w248
          tunnel: w244 -> [w257 w270 w272 w281 w292 w295 w298 w315 w333 w343]
          tunnel: [w256 w270 w272 w280 w292 w295 w298 w315 w333 w343] -> w243
          tunnel: [_ _ _ _ _ _ _ _ w332 _] -> w242
          tunnel: w240 -> [_ _ _ w277 _ _ _ w314 w331 _]
          tunnel: w237 -> [w258 _ _ _ _ _ _ w312 w326 _]
          frame "Initialize" {
            w251 = "Started Dashboard" ("Initial Message")
            # "Initialize - Any operation that needs to be done before the module can receive messages. Synchronize Caller Events.vi will inform Start Module.vi that the module has launched and is ready to receive messages. Module Did Init.vi will broadcast that the module initialized."
            n176 = call "Synchronize Caller Events.vi"("error in (no error)"=w267, "Singleton Module Admin in"=w258) -> ("error out"=w266:errorcluster, "Singleton Module Admin out"=w253:refnum<class "Delacor_lib_QMH_Module Admin.lvclass">)  [unwired: 8 in]
            n177 = property class="Module Admin"(reference=w253) -> ("Accessors:External Launch"=w262:bool)  [unwired: 1 in, 2 out]
            n178 = Select(t=T13."Hidden" ("State"), s=w262, f=T13."Standard" ("State")) -> (s? t:f=w259:T13)
            n179 = call "Module Name--constant.vi"() -> ("Module Name"=w254:string)  [unwired: 11 in]
            n180 = call "Module Name--constant.vi"() -> ("Module Name"=w265:string)  [unwired: 11 in]
            n181 = property class="VI"("Front Panel.Title"=w265) -> (reference out=w264:refnum<vi>, error out=w269:errorcluster)  [unwired: 2 in]
            n182 = call "Module Did Init.vi"("error in (no error)"=w266, "Initialized?"=TRUE, "Origin"=w254) -> ("error out"=w250:errorcluster)  [unwired: 8 in]
            n183 = invoke class="VI" method="FP.Open"(reference=w264, error in=w269, "State"=w259) -> (reference out=w263:refnum<vi>, error out=w268:errorcluster)  [unwired: 2 in, 3 out]
            n184 = call "Get Module Execution Status.vi"("error in (no error)"=w250) -> ("error out"=w249:errorcluster)  [unwired: 10 in]
            n185 = invoke class="VI" method="FP.Center"(reference=w263, error in=w268) -> ()  [unwired: 1 in, 3 out]
            n186 = property on="Pane" class="Pane"("Origin"=T18 {"Horizontal"=0, "Vertical"=0}) -> ()  [unwired: 2 in, 2 out]
            n187 = Bundle By Name(cluster=w257, "Status"=w251) -> (w256:T12)
            "Status" <- w251
          }
          frame "--- Module Specific ---" {
            # "Separator -- The following cases handle messages specific to this Module."
          }
          frame "---Copy This Frame---" {
            # "Duplicate this frame when creating new messages.  Change this comment in the duplicated frame to describe this message."
            n188 = Merge Errors(w274) -> (w273:errorcluster)
          }
          frame "Update Spectrum" {
            # "Write the image to the module data cluster"
            n189 = Variant To Data(error in=w283, type=T15 {"Image"=[]} ("Update Image Argument"), Variant=w277) -> (data=w276:T15, error out=w279:errorcluster)
            n190 = Unbundle By Name(w276) -> ("Image"=w275:u16[][])
            n191 = Bundle By Name(cluster=w281, "Image"=w275) -> (w280:T12)
            n192 = Merge Errors(w279) -> (w282:errorcluster)
          }
          frame "Display Spectrum" {
            # "convert to double, otherwise we get an overflow"
            # "Display the spectrum with appropriate x and y values"
            n193 = Unbundle By Name(w292) -> ("Image"=w291:u16[][])
            "Spectrum Graph" <- w291
            n194 = Transpose 2D Array(2D array=w291) -> (transposed array=→"CCD Image":u16[][])
            n195 = To Double Precision Float(number=w291) -> (double precision float=w286:dbl[][])
            n196 = Array Size(array=w291) -> (size(s)=w290:i32[])
            n197 = Add Array Elements(numeric array=w286) -> (sum=w285:dbl)
            n198 = Multiply Array Elements(1:w290) -> (0:w288:i32)
            n199 = To Double Precision Float(number=w288) -> (double precision float=w287:dbl)
            n200 = Divide(x=w285, y=w287) -> (x/y=→"Waveform Chart":dbl)
            n201 = Merge Errors(w294) -> (w293:errorcluster)
          }
          frame "--- Exit and Error Handling---" {
            # "Separator - The following cases handle errors and exit messages."
          }
          frame "Simulate MHL Error" {
            # "#DQMH_HowTo The 'Simulate MHL Error' button  illustrates how the MHL handles errors. This event is instructional in nature and can be removed."
            # "Simulate an error occurring at the MHL"
            n202 = call "Module Name--constant.vi"() -> ("Module Name"=w297:string)  [unwired: 11 in]
            n203 = xnode "Error Ring"("parameter 0"=w297) -> ("error out"=w299:errorcluster)
            n204 = Merge Errors(w301, w299) -> (w300:errorcluster)
          }
          frame "Error" {
            # "#CodeRecommended - If you ever change the name of this \"Error\" message, you'll need to update the name in the Check Loop Error.vi as well."
            # "#CodeRecommended - If the module is running in standalone mode (External Launch = FALSE), this code will pop up an error dialog and call the 'Exit' message if an error occurs. Add more fine-grained error handling here."
            # "Error - Check the error message data and respond accordingly. This message is sent by the \"Error Handler\" VIs at the end of each loop in this application."
            n205 = property class="Module Admin"(reference=w312) -> ("Accessors:External Launch"=w311:bool)  [unwired: 1 in, 2 out]
            n206 = Variant To Data(error in=w319, type=errorcluster {"status"=FALSE, "code"=0, "source"=""} ("error constant"), Variant=w314) -> (data=w320:errorcluster, error out=w317:errorcluster)
            n207 = call "Module Name--constant.vi"() -> ("Module Name"=w310:string)  [unwired: 11 in]
            n208 = call "Error Reported.vi"("Additional Information"=w310, "Error"=w320) -> ()  [unwired: 9 in, 1 out]
            n209 = case shown="False" w311 {
              tunnel: [w325 _] -> w316
              tunnel: w313 -> [w323 _]
              tunnel: w320 -> [w324 _]
              frame False {
                # "If the module is running standalone, then pop up an error dialog and call the \"Exit\" message."
                n210 = call <vilib>:"Simple Error Handler.vi"("error in (no error)"=w324) -> ()  [unwired: 4 in, 5 out]
                n211 = call-poly <vilib>:"Delacor_lib_QMH_Enqueue Message (poly).vi"("Priority Message? (F)"=TRUE, "Message"="Exit", "Message Queue in"=w323) -> ("error out"=w325:errorcluster)  [unwired: 7 in, 1 out]
              }
              frame True {
                # "If the module was launched externally, calling the Error Reported broadcast VI is the only action performed by the \"Error\" message. The module's caller can then process the error appropriately."
              }
            }
            n212 = Merge Errors(w317, w316) -> (w309:errorcluster)
            n213 = call <vilib>:"Simple Error Handler.vi"("error in (no error)"=w309) -> ()  [unwired: 4 in, 5 out]
          }
          frame "Exit" {
            w330 = 91  # 91: not all Exit messages will have an argument
            w332 = TRUE  # Stop the VI
            # "Release the message queue reference"
            # "#CodeNeeded - Add any required cleanup code here"
            # "Exit - Exit the application."
            n214 = Variant To Data(error in=w340, type=T17 {"Origin"="", "Exit via Stop Module Req?"=FALSE, "Wait for Module to stop?"=FALSE} ("Stop Argument"), Variant=w331) -> (data=w328:T17, error out=w336:errorcluster)
            n215 = call <vilib>:"Clear Errors.vi"("error in (no error)"=w336, "specific error code to clear (0: all)"=w330) -> ("error out"=w339:errorcluster)  [unwired: 4 in, 1 out]
            n216 = control-ref of="This VI"() -> (w327:refnum<vi>)
            n217 = call-dynamic "Delacor_lib_QMH_Release Message Queue.vi"("error in (no error)"=w339, "Message Queue"=w334) -> ("error out"=w338:errorcluster)  [unwired: 9 in]
            n218 = call "Handle Exit.vi"("Stop Argument"=w328, "Admin in"=w326, "VI reference"=w327) -> ("error out"=w335:errorcluster)  [unwired: 7 in, 1 out]
            n219 = Merge Errors(w338, w335) -> (w337:errorcluster)
            n220 = call "Stop Module.vi"() -> ()  [unwired: 11 in, 1 out]
          }
          frame Default {
            # "'Default' case only runs if there is a message that isn't defined in any of the other cases.  Output a programming error."
            n221 = call "Module Name--constant.vi"() -> ("Module Name"=w341:string)  [unwired: 11 in]
            n222 = xnode "Error Ring"("parameter 0"=w342, "parameter 1"=w341) -> ("error out"=w346:errorcluster)
            n223 = Merge Errors(w344, w346) -> (w345:errorcluster)
          }
        }
        n224 = call-dynamic "Delacor_lib_QMH_Error Handler - Message Handling Loop.vi"("error in (no error)"=w248, "Message Queue in"=w238) -> ("dup error in"=w245:errorcluster)  [unwired: 8 in, 1 out]
      }
    }
    frame Error {
      # "Synchronize Caller Events.vi will inform Start Module.vi that the module has launched and will let the code calling Start Module.vi register for broadcasts and would permit the caller receive the broadcast that an error occurred at launch time."
      n225 = call-dynamic "Delacor_lib_QMH_Release Message Queue.vi"("error in (no error)"=w357, "Message Queue"=w355) -> ("error out"=w356:errorcluster)  [unwired: 9 in]
      n226 = call "Synchronize Caller Events.vi"("Singleton Module Admin in"=w358) -> ("error out"=w363:errorcluster)  [unwired: 9 in, 1 out]
      n227 = call "Module Name--constant.vi"() -> ("Module Name"=w361:string)  [unwired: 11 in]
      n228 = Format Into String(format string="An error occurred during initialization. %s is no longer running.", w361) -> (resulting string=w359:string)  [unwired: 2 in, 1 out]
      n229 = Merge Errors(w356, w363) -> (w364:errorcluster)
      n230 = call "Error Reported.vi"("Additional Information"=w359, "Error"=w364) -> ()  [unwired: 9 in, 1 out]
    }
  }
  n231 = Merge Errors(w18, w21) -> (w17:errorcluster)
  n232 = call "Close Module.vi"("error in (no error)"=w17, "Module Admin in"=w12) -> ("error out"=w19:errorcluster, "External Launch"=w5:bool, "Module Admin out"=w6:refnum<class "Delacor_lib_QMH_Module Admin.lvclass">)  [unwired: 7 in]
  n233 = Unregister For Events(event registration refnum=w11, error in=w19) -> (error out=w16:errorcluster)
  n234 = case "External Launch?" shown="True" w5 {
    tunnel: w16 -> [_ w365]
    frame False {
    }
    frame True {
      n235 = case shown="No Error" w365 {
        frame No Error {
          n236 = invoke class="VI" method="FP.Close"() -> ()  [unwired: 3 in, 3 out]
        }
        frame Error {
          n237 = invoke class="VI" method="FP.Open"("Activate"=TRUE ("Activate?")) -> ()  [unwired: 4 in, 5 out]
        }
      }
    }
  }
  n238 = local write "Module Admin"(w6) -> ()
